vi "Get Current Session.vi"(8 "error in (no error)":errorcluster, 11 "Authentication Service":refnum<class "Authentication Service.lvclass">) -> (0 "error out":errorcluster, 3 "Current Session":refnum<class "Session.lvclass">)   [LabVIEW 2026, in "Authentication Service.lvclass"]
uses:
  Authentication Service.lvclass
  Authentication Service.lvclass/Authentication Service.ctl
  Domain/Session/Session.lvclass
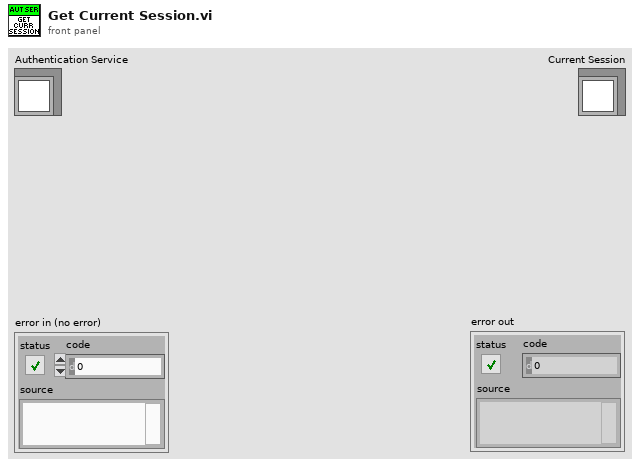
[diagram p1: front panel]
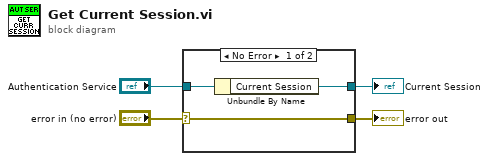
[diagram p0: block diagram]
diagram:
  n1 = case shown="No Error" "error in (no error)" {
    selector: "error in (no error)" -> [w5 w8]
    tunnel: "Authentication Service" -> [w7 _]
    tunnel: [w6 _] -> w3
    tunnel: [w5 w8] -> w1
    frame No Error {
      n2 = Unbundle By Name(w7) -> ("Current Session"=w6:refnum<class "Session.lvclass">)
    }
    frame Error {
    }
  }
  "Current Session" <- w3
  "error out" <- w1
